vi "ScalingFactorProperty.vi"(7 "Write?":bool, 8 "error in (no error)":errorcluster, 10 "Value in":sgl, 11 "QR Code Detector in":refnum<class "WeChat QR Code Detector.lvclass">) -> (0 "error out":errorcluster, 3 "Value out":sgl)   [LabVIEW 2020, in "feature_detection.lvlib" / "WeChat QR Code Detector.lvclass"]
uses:
  WeChat QR Code Detector.lvclass
  WeChat QR Code Detector.lvclass/WeChat QR Code Detector.ctl
  common/common.lvlib
  common/bin/gartoolkit_dnn_32-1.dll
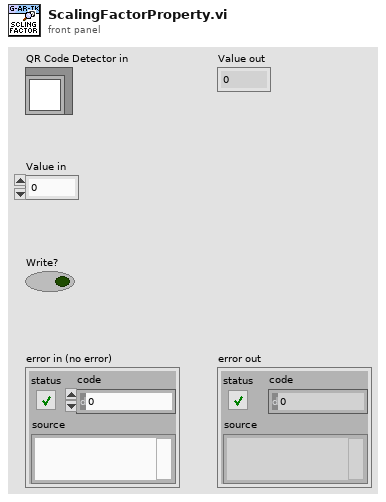
[diagram p1: front panel]
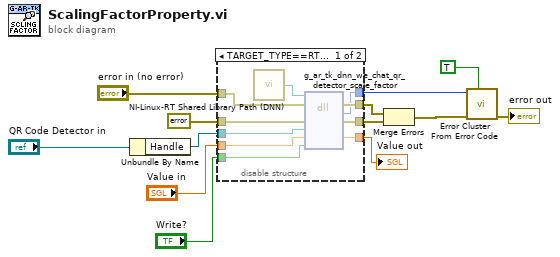
[diagram p0: block diagram]
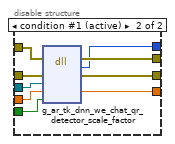
[diagram p2: hidden frame]
diagram:
  n1 = Unbundle By Name("QR Code Detector in") -> ("Handle"=w9:refnum<data-value>)
  n2 = disable-structure shown="TARGET_TYPE==RT&&OS==Linux" {
    disable-tunnel: "error in (no error)" -> [w22 w32]
    disable-tunnel: errorcluster {"status"=FALSE, "code"=0, "source"=""} ("error constant") -> [w21 w31]
    disable-tunnel: w9 -> [w20 w30]
    disable-tunnel: "Value in" -> [w19 w29]
    disable-tunnel: "Write?" -> [w18 w28]
    disable-tunnel: [w17 w27] -> w6
    disable-tunnel: [w15 w26] -> w5
    disable-tunnel: [w16 w25] -> w4
    disable-tunnel: [w14 w24] -> w1
    frame condition #0 {
      n3 = call "NI-Linux-RT Shared Library Path (DNN).vi"() -> ("Path"=w23:path)
      n4 = dll-call lib="?" fn="g_ar_tk_dnn_we_chat_qr_detector_scale_factor" ("g_ar_toolkit.*.*:g_ar_tk_capture_context_create")(path in=w23, error in=w22, "error_cluster"=w21, "Detector_EDVR"=w20, "Value"=w19, "Write"=w18) -> (error out=w17:errorcluster, "return type"=w15:i32, "error_cluster"=w14:errorcluster, "Value"=w16:sgl)  [unwired: 3 in, 1 out]
    }
    frame condition #1 (active) {
      n5 = dll-call lib="C:/serenial/lib/g-augmented-reality-toolkit/LabVIEW/common/bin/gartoolkit_dnn_*-1.*" fn="g_ar_tk_dnn_we_chat_qr_detector_scale_factor" ("g_ar_toolkit.*.*:g_ar_tk_capture_context_create")(error in=w32, "error_cluster"=w31, "Detector_EDVR"=w30, "Value"=w29, "Write"=w28) -> (error out=w27:errorcluster, w26:i32, "error_cluster"=w24:errorcluster, "Value"=w25:sgl)  [unwired: 4 in, 1 out]
    }
  }
  "Value out" <- w4
  n6 = Merge Errors(w6, w1) -> (w2:errorcluster)
  n7 = call <vilib>:"Error Cluster From Error Code.vi"("show call chain? (False)"=TRUE, "error in (no error)"=w2, "error code (0)"=w5) -> ("error out"=→"error out":errorcluster)  [unwired: 6 in]
